vi "Query Max Current Limit.vi"(8 "error in (no error)":errorcluster, 11 "VISA resource name":refnum<visa-resource-name>) -> (0 "error out":errorcluster, 2 "Max Current Limit":dbl format="%.2p", 3 "VISA resource name out":refnum<visa-resource-name>)   [LabVIEW 2020, in "Agilent E364X Series.lvlib"]
doc: "This VI returns the maximum programmable current limit that the power supply accepts for the output range to which the power supply is currently configured."
uses:
  Agilent E364X Series.lvlib
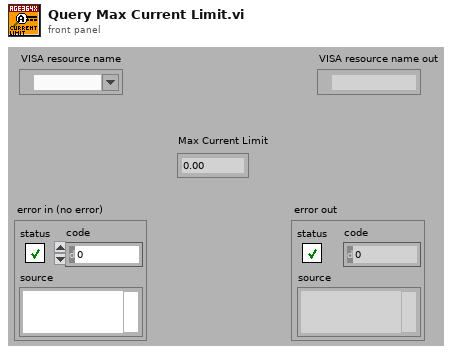
[diagram p1: front panel]
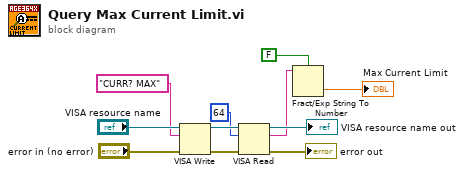
[diagram p0: block diagram]
diagram:
  n1 = VISA Write(VISA resource name="VISA resource name", write buffer="CURR? MAX", error in (no error)="error in (no error)") -> (VISA resource name out=w9:refnum<visa-resource-name>, error out=w8:errorcluster)  [unwired: 1 out]
  n2 = VISA Read(VISA resource name=w9, byte count=u32 64, error in (no error)=w8) -> (VISA resource name out=→"VISA resource name out":refnum<visa-resource-name>, read buffer=w4:string, error out=→"error out":errorcluster)  [unwired: 1 out]
  n3 = Fract/Exp String To Number(use system decimal point (T)=FALSE, string=w4) -> (number=→"Max Current Limit":dbl)  [unwired: 2 in, 1 out]
